vi "HCC Split Voltage and Current Agilent.vi"(8 "Error In":errorcluster, 10 "Input Agilent Array":dbl[](array[numeric]), 11 "Voltage Indexes":i32[](array[numeric])) -> (0 "Error Out":errorcluster, 2 "Voltage Array":dbl[](array[numeric]), 3 "Current Array":dbl[](array[numeric]))   [LabVIEW 2016]
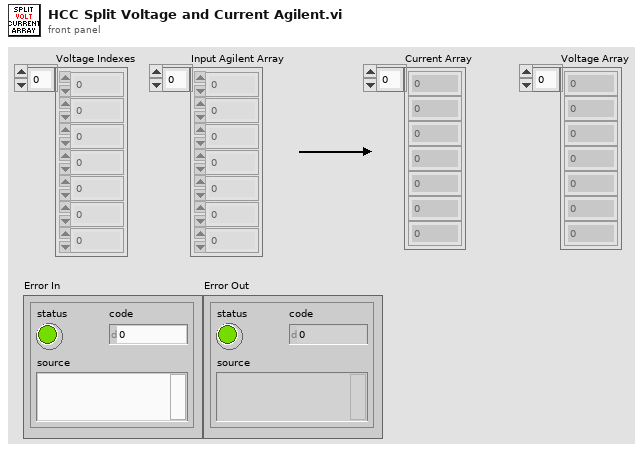
[diagram p1: front panel]
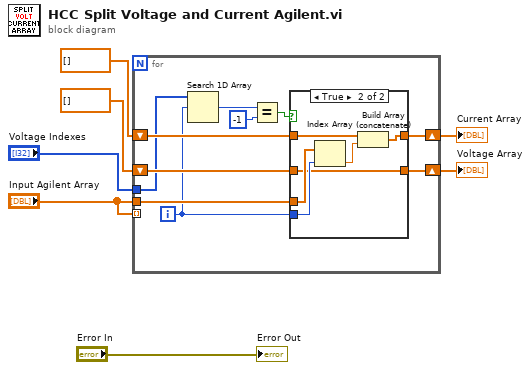
[diagram p0: block diagram]
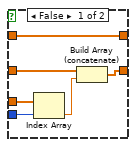
[diagram p2: hidden frame]
diagram:
  n1 = for {
    tunnel: "Input Agilent Array" -> [_] mode=indexing
    tunnel: "Input Agilent Array" -> [w14]
    shift-right: [w15] -> w6
    shift-left: dbl[] [] -> [w16]
    shift-right: [w11] -> w7
    shift-left: dbl[] [] -> [w12]
    tunnel: "Voltage Indexes" -> [w10]
    i -> [w8]
    n2 = Search 1D Array(1D array=w10, element=w8) -> (index of element=w13:i32)  [unwired: 1 in]
    n3 = Equal?(x=w13, y=-1) -> (x = y?=w9:bool)
    n4 = case shown="True" w9 {
      tunnel: w16 -> [w23 w29]
      tunnel: [w23 w28] -> w15
      tunnel: w14 -> [w19 w27]
      tunnel: w8 -> [w20 w26]
      tunnel: w12 -> [w21 w24]
      tunnel: [w18 w24] -> w11
      frame False {
        n5 = Index Array(array=w19, index=w20) -> (element=w22:dbl)
        n6 = Build Array (concatenate)(w21, w22) -> (w18:dbl[])
      }
      frame True {
        n7 = Index Array(array=w27, index=w26) -> (element=w25:dbl)
        n8 = Build Array (concatenate)(w29, w25) -> (w28:dbl[])
      }
    }
  }
  "Voltage Array" <- w7
  "Current Array" <- w6
  "Error Out" <- "Error In"
